vi "Find Red Pitayas.vi"(6 "Timeout":i32=100, 7 "Logic tags":u16[](array[numeric])=[101, 102, 104, 105, 107, 108, 109, 111, 112, 113, 114, 152, 154, 155, 157, 158, 159, 164, 169], 8 "Error In":errorcluster, 9 "End address":i32=120, 10 "Start address":i32=100, 11 "Subnet":string="192.168.1") -> (0 "Error Out":errorcluster, 1 "Addresses":string[](array[string]), 2 "Device names":string[](array[string]), 3 "Modules":i32[](array[numeric]), 4 "DDS modula out":i64[](array[numeric])=[101, 102], 5 "Logic tags out":u16[](array[numeric])=[101, 102])   [LabVIEW 2024, in "Red Pitaya Digitizer.lvclass"]
uses:
  Red Pitaya Digitizer.lvclass
  Red Pitaya Digitizer.lvclass/Red Pitaya Digitizer.ctl
  RP Core/RP Communicator/RP Communicator.lvclass
panel:
  out "ID tags out 2":u32[](array[numeric])=[101, 102]
  out "Logic tags out 2":u16[](array[numeric])=[101, 102]
  out "Last address byte":i32[](array[numeric])
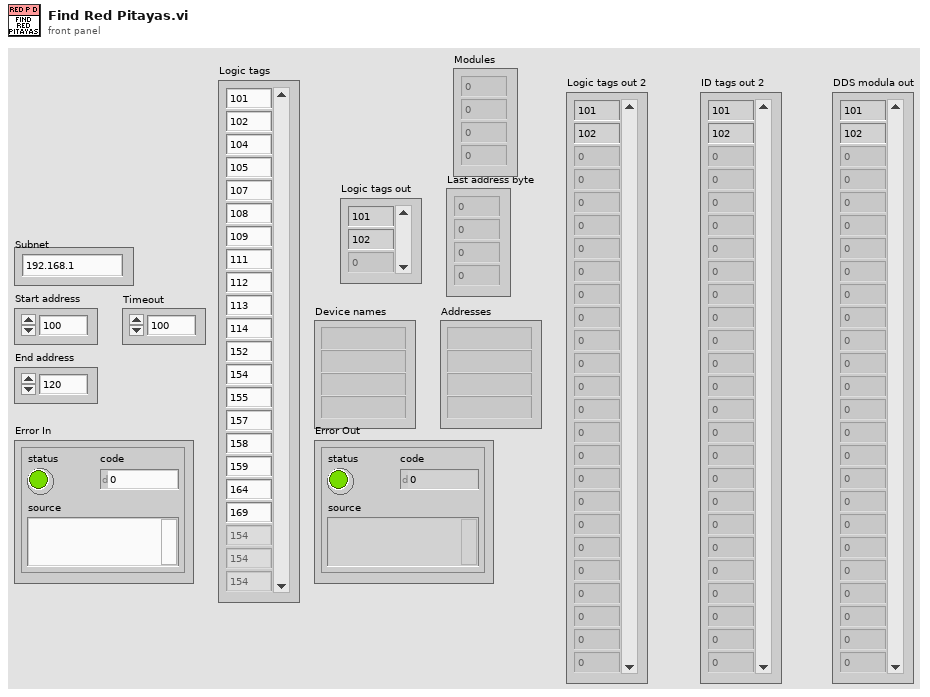
[diagram p1: front panel]
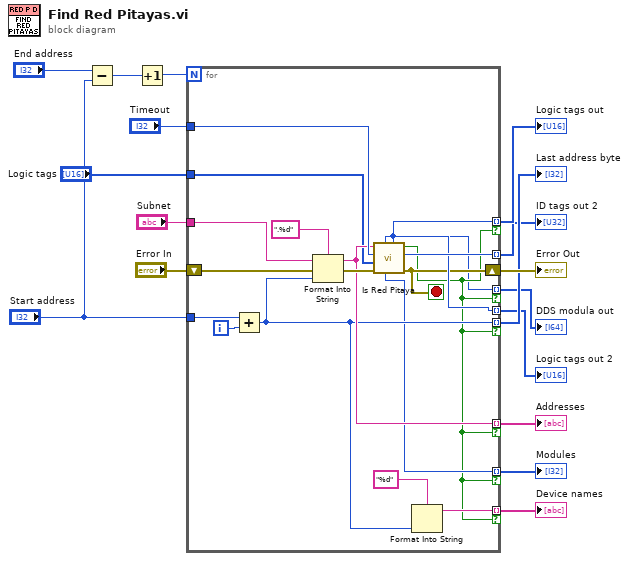
[diagram p0: block diagram]
diagram:
  n1 = Subtract(x="End address", y="Start address") -> (x-y=w16:i32)
  n2 = Increment(x=w16) -> (x+1=w15:i32)
  n3 = for {
    N: w15 -> [_]
    tunnel: "Start address" -> [w33]
    tunnel: "Subnet" -> [w31]
    tunnel: "Timeout" -> [w30]
    tunnel: [w29] -> w10 mode=indexing if=w19
    shift-right: [w20] -> w8
    shift-left: "Error In" -> [w28]
    tunnel: [w26] -> w9 mode=indexing if=w19
    tunnel: "Logic tags" -> [w21]
    tunnel: [w23] -> w6 mode=indexing if=w19
    tunnel: [w25] -> w5 mode=indexing if=w19
    tunnel: [w24] -> w3 mode=indexing
    tunnel: [w23] -> w4 mode=indexing
    tunnel: [w22] -> w2 mode=indexing if=w19
    tunnel: [w18] -> w1 mode=indexing if=w19
    i -> [w34]
    stop <- w20 stop-if-true
    n4 = Add(x=w33, y=w34) -> (x+y=w25:i32)
    n5 = Format Into String(format string=".%d", initial string=w31, error in=w28, w25) -> (resulting string=w29:string, error out=w35:errorcluster)
    n6 = call "Is Red Pitaya.vi"("Error In"=w35, "Acceptable logic tags"=w21, "Timeout"=w30, "Server address"=w29) -> ("Error Out"=w20:errorcluster, "IDN response"=w24:u32, "Red Pitaya"=w19:bool, "Logic tag out"=w23:u16, "Module"=w22:i32, "DDS modulus"=w18:i64)  [unwired: 2 out]
    n7 = Format Into String(format string="%d", w25) -> (resulting string=w26:string)  [unwired: 2 in, 1 out]
  }
  "Device names" <- w9
  "Error Out" <- w8
  "Addresses" <- w10
  "Logic tags out" <- w6
  "Last address byte" <- w5
  "Logic tags out 2" <- w4
  "ID tags out 2" <- w3
  "Modules" <- w2
  "DDS modula out" <- w1
